vi "Read NChan NSamp 1D Waveform.vi"(8 "error in (no error)":errorcluster, 9 "timeout [s]":dbl=-1.0, 10 "number of samples per channel":i32=1000, 11 "MicroDAQ.lvlib:Analog Input.lvclass":refnum<class "Analog Input.lvclass">) -> (0 "error out":errorcluster, 2 "Values":waveform(dbl)[](array[waveform]), 3 "MicroDAQ.lvlib:Analog Input.lvclass out":refnum<class "Analog Input.lvclass">)   [LabVIEW 2009, in "MicroDAQ.lvlib" / "Analog Input.lvclass"]
doc: "Reads a waveform from each channel."
uses:
  <instrlib>/MicroDAQ/Channel/Analog Input/Analog Input.lvclass
  <instrlib>/MicroDAQ/Channel/Analog Input/Analog Input.lvclass/Analog Input.ctl
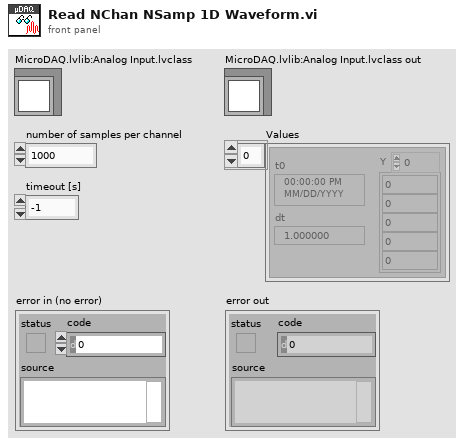
[diagram p1: front panel]
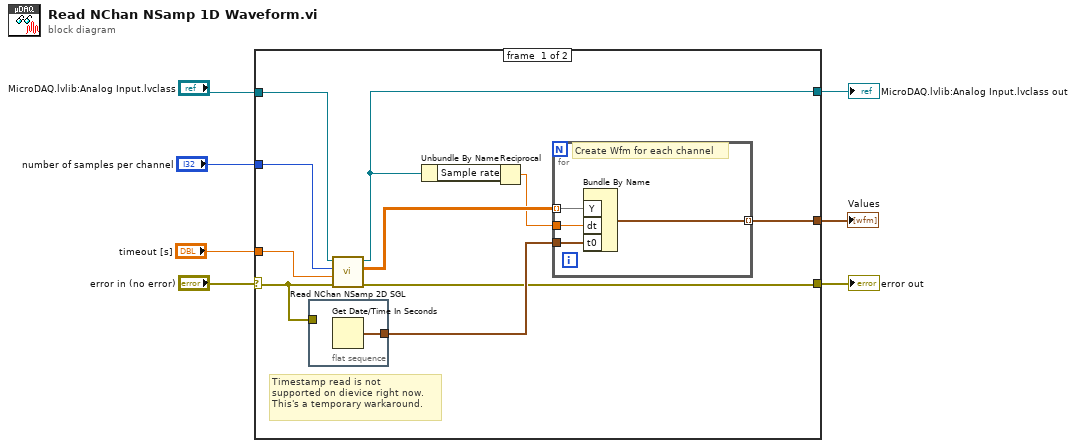
[diagram p0: block diagram]
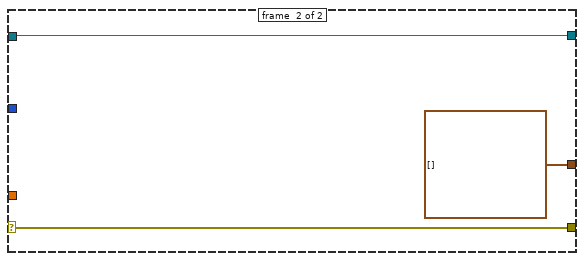
[diagram p2: hidden frame]
diagram:
  n1 = case shown="No Error" "error in (no error)" {
    selector: "error in (no error)" -> [w18 w25]
    tunnel: [w9 w25] -> w6
    tunnel: [w14 w26] -> w5
    tunnel: "number of samples per channel" -> [w16 _]
    tunnel: "MicroDAQ.lvlib:Analog Input.lvclass" -> [w17 w26]
    tunnel: [w10 waveform(dbl)[] []] -> w2
    tunnel: "timeout [s]" -> [w8 _]
    frame #0 {
      # "Timestamp read is not \nsupported on dievice right now.\nThis's a temporary warkaround."
      n2 = flat-sequence {
        tunnel: w18 -> [_]
        tunnel: [w23] -> w11
        frame #0 {
          n3 = Get Date/Time In Seconds() -> (seconds since 1Jan1904=w23:timestamp)
        }
      }
      n4 = call <instrlib>:"Read NChan NSamp 2D SGL.vi"("error in (no error)"=w18, "timeout [s]"=w8, "number of samples per channel"=w16, "MicroDAQ.lvlib:Analog Input.lvclass"=w17) -> ("error out"=w9:errorcluster, "Values"=w13:dbl[][], "MicroDAQ.lvlib:Analog Input.lvclass out"=w14:refnum<class "Analog Input.lvclass">)  [unwired: 4 in, 1 out]
      n5 = Unbundle By Name(w14) -> ("Sample rate"=w15:sgl)
      n6 = Reciprocal(x=w15) -> (1/x=w12:sgl)
      n7 = for {
        tunnel: w13 -> [w22] mode=indexing
        tunnel: w12 -> [w21]
        tunnel: w11 -> [w20]
        tunnel: [w19] -> w10 mode=indexing
        # "Create Wfm for each channel"
        n8 = Bundle By Name("Y"=w22, "dt"=w21, "t0"=w20) -> (w19:waveform(dbl))  [unwired: 1 in]
      }
    }
    frame #1 {
    }
  }
  "error out" <- w6
  "MicroDAQ.lvlib:Analog Input.lvclass out" <- w5
  "Values" <- w2
